vi "Rinocloud_simulator (SubVI).vi"(0 "x timestamps in":string[](array[string]), 1 "x axis in":dbl[](array[numeric]), 5 "x native timestamp in":timestamp[](array[timestamp]), 7 "date time rec":T1, 9 "z axis in":dbl[](array[numeric]), 12 "2D data in":dbl[][](array[numeric])) -> (3 "x axis out":dbl[](array[numeric]), 4 "x timestamps out":string[](array[string]), 6 "x native timestamp out":timestamp[](array[timestamp]), 8 "z axis out":dbl[](array[numeric]), 10 "Array 2":dbl[](array[numeric]), 13 "Array":dbl[](array[numeric]), 14 "2D data out":dbl[][](array[numeric]))   [LabVIEW 2013, in "Rinocloud Library.lvlib"]
uses:
  <vilib>/Utility/miscctls.llb/LVDateTimeRec.ctl
  Rinocloud Library.lvlib
  <vilib>/Analysis/NI_AALBase.lvlib
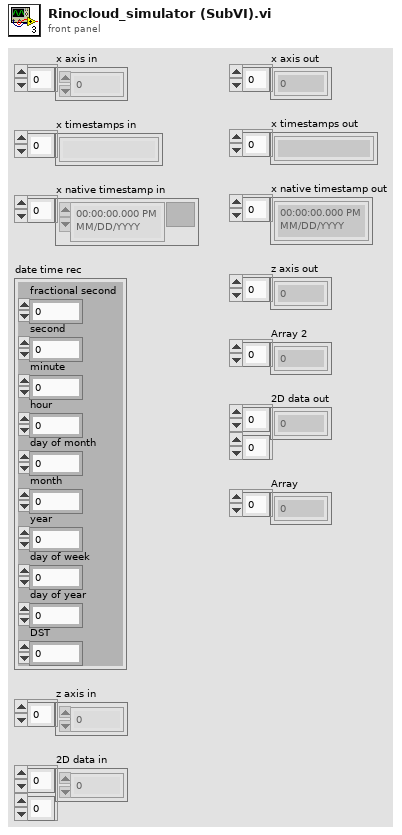
[diagram p1: front panel]
types:
  T1 = typedef "LVDateTimeRec.ctl" = cluster{"fractional second":dbl, "second":i32, "minute":i32, "hour":i32, "day of month":i32, "month":i32, "year":i32, "day of week":i32, "day of year":i32, "DST":i32}
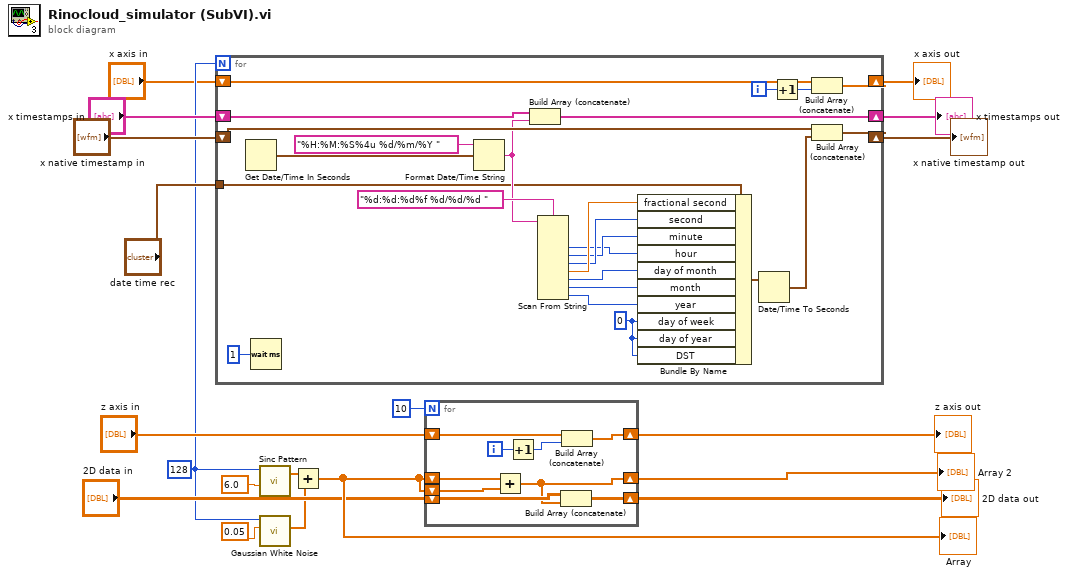
[diagram p0: block diagram]
diagram:
  w6 = 128 ("samples")
  n1 = for {
    N: w6 -> [_]
    shift-right: [w42] -> w12
    shift-left: "x axis in" -> [w43]
    shift-right: [w37] -> w16
    shift-left: "x timestamps in" -> [w38]
    shift-right: [w33] -> w18
    shift-left: "x native timestamp in" -> [w35]
    tunnel: "date time rec" -> [w30]
    i -> [w41]
    w22 = 0 ("day of week")
    n2 = Get Date/Time In Seconds() -> (seconds since 1Jan1904=w34:timestamp)
    n3 = Wait (ms)(milliseconds to wait=u32 1) -> ()  [unwired: 1 out]
    n4 = Format Date/Time String(time format string (%c)="%H:%M:%S%4u %d/%m/%Y ", seconds (now)=w34) -> (date/time string=w31:string)  [unwired: 1 in]
    n5 = Build Array (concatenate)(w38, w31) -> (w37:string[])
    n6 = Scan From String(format string="%d:%d:%d%f %d/%d/%d " ("time format string (%c)"), input string=w31) -> (output 1=w26:i32, output 2=w27:i32, output 3=w28:i32, output 4=w29:dbl, output 5=w25:i32, output 6=w24:i32, output 7=w23:i32)  [unwired: 9 in, 3 out]
    n7 = Bundle By Name(cluster=w30, "fractional second"=w29, "second"=w28, "minute"=w27, "hour"=w26, "day of month"=w25, "month"=w24, "year"=w23, "day of week"=w22, "day of year"=w22, "DST"=w22) -> (w21:T1)
    n8 = Date/Time To Seconds(2:w21) -> (0:w20:timestamp)  [unwired: 1 in]
    n9 = Increment(x=w41) -> (x+1=w40:i32)
    n10 = Build Array (concatenate)(w43, w40) -> (w42:dbl[])
    n11 = Build Array (concatenate)(w35, w20) -> (w33:timestamp[])
  }
  "x native timestamp out" <- w18
  "x timestamps out" <- w16
  "x axis out" <- w12
  n12 = call <vilib>:"Sinc Pattern.vi"("delay"=6.0, "samples"=w6) -> ("Sinc Pattern"=w4:dbl[])  [unwired: 2 in, 1 out]
  n13 = call <vilib>:"Gaussian White Noise.vi"("standard deviation"=0.05, "samples"=w6) -> ("Gaussian noise pattern"=w3:dbl[])  [unwired: 8 in, 1 out]
  n14 = Add(x=w4, y=w3) -> (x+y=w11:dbl[])
  "Array" <- w11
  n15 = for {
    N: 10 -> [_]
    shift-right: [w51] -> w9
    shift-left: "2D data in" -> [w52]
    shift-right: [w49] -> w10
    shift-left: w11 -> [w48]
    shift-left: w11 -> [w50]
    shift-right: [w46] -> w14
    shift-left: "z axis in" -> [w45]
    i -> [w44]
    n16 = Add(x=w48, y=w50) -> (x+y=w49:dbl[])
    n17 = Increment(x=w44) -> (x+1=w47:i32)
    n18 = Build Array (concatenate)(w52, w49) -> (w51:dbl[][])
    n19 = Build Array (concatenate)(w45, w47) -> (w46:dbl[])
  }
  "z axis out" <- w14
  "Array 2" <- w10
  "2D data out" <- w9
